vi "Initialize_DBL.vi"(8 "error in (no error)":errorcluster, 9 "Radius":dbl, 10 "Angle (degrees)":dbl) -> (0 "error out":errorcluster, 3 "PolarVector out":refnum<class "PolarVector.lvclass">)   [LabVIEW 2013, in "PolarVector.lvclass"]
doc: "Takes in a DBL for both the angle and the radius and outputs a PolarVector object."
uses:
  PolarVector.lvclass
  Angles/Angle/Angle.lvclass
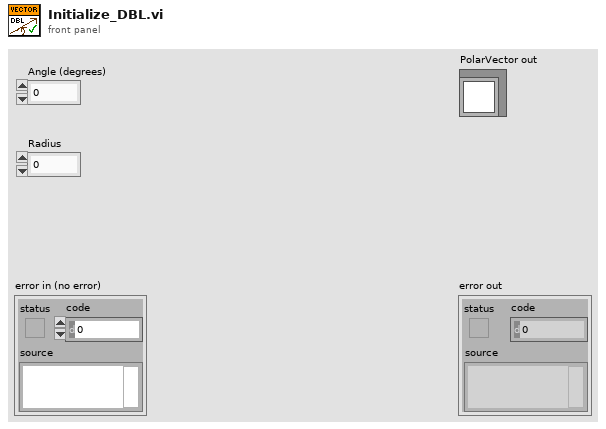
[diagram p1: front panel]
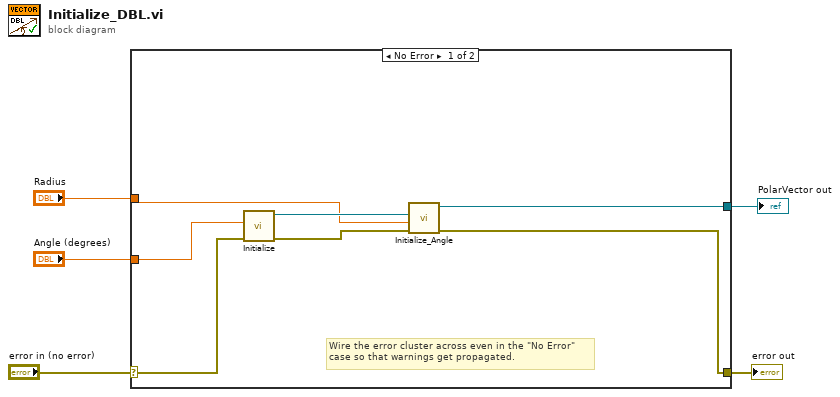
[diagram p0: block diagram]
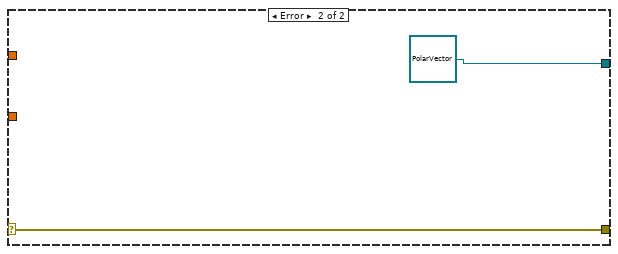
[diagram p2: hidden frame]
diagram:
  n1 = case shown="No Error" "error in (no error)" {
    selector: "error in (no error)" -> [w11 w14]
    tunnel: [w8 w14] -> w4
    tunnel: "Angle (degrees)" -> [w12 _]
    tunnel: "Radius" -> [w6 _]
    tunnel: [w7 refnum<class "PolarVector.lvclass"> refnum ("PolarVector out")] -> w1
    frame No Error {
      # "Wire the error cluster across even in the \"No Error\"\ncase so that warnings get propagated."
      n2 = call "Initialize.vi"("error in (no error)"=w11, "Input Angle (Deg.)"=w12) -> ("error out"=w9:errorcluster, "Angle out"=w10:refnum<class "Angle.lvclass">)  [unwired: 8 in]
      n3 = call "Initialize_Angle.vi"("error in (no error)"=w9, "Radius"=w6, "Angle.lvclass"=w10) -> ("error out"=w8:errorcluster, "PolarVector out"=w7:refnum<class "PolarVector.lvclass">)  [unwired: 7 in]
    }
    frame Error {
    }
  }
  "error out" <- w4
  "PolarVector out" <- w1
